vi "TestArrow.vi"() -> ()   [LabVIEW 2018]
uses:
  <vilib>/userdefined/High Color/IMAQdx.ctl
  <vilib>/vision/driver/NI_Vision_Acquisition_Software.lvlib
  <resource>/objmgr/imaqdx.rc
panel:
  in  "Slide":dbl(slide) scale=-1.0..1.0
  out "x-y":u32
  in  "stop":bool
  out "Image":T1(plugin-control)
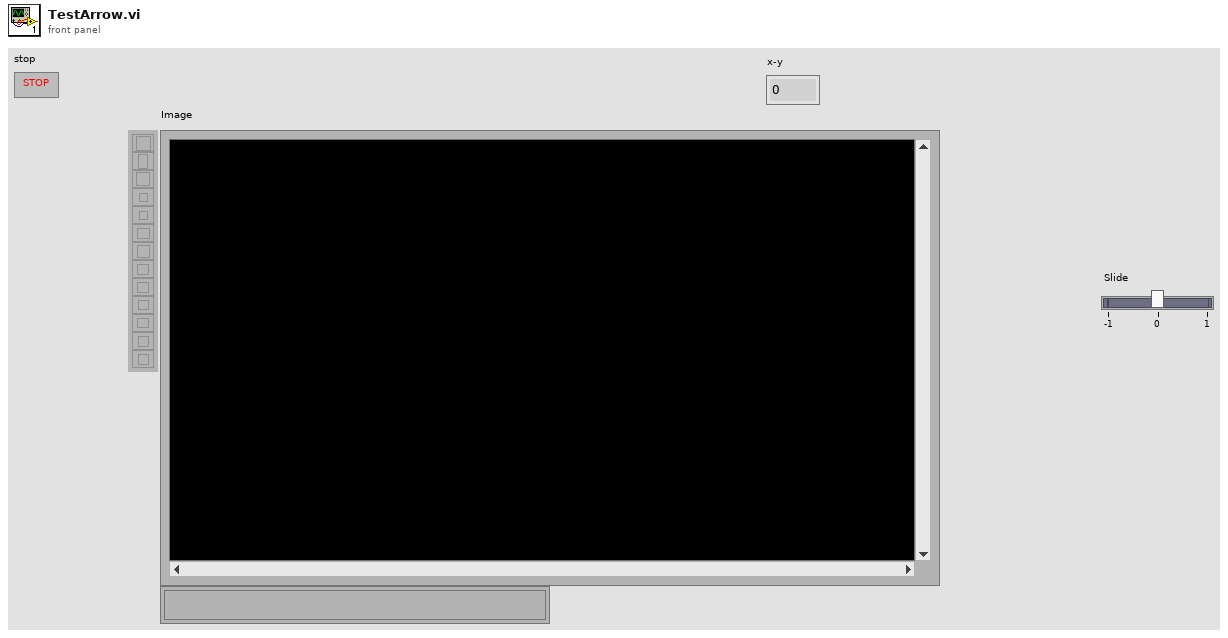
[diagram p1: front panel]
types:
  T1 = typedef "IMAQ Image.ctl" = refnum<image>
  T2 = typedef "IMAQdx.ctl" = refnum<k21>
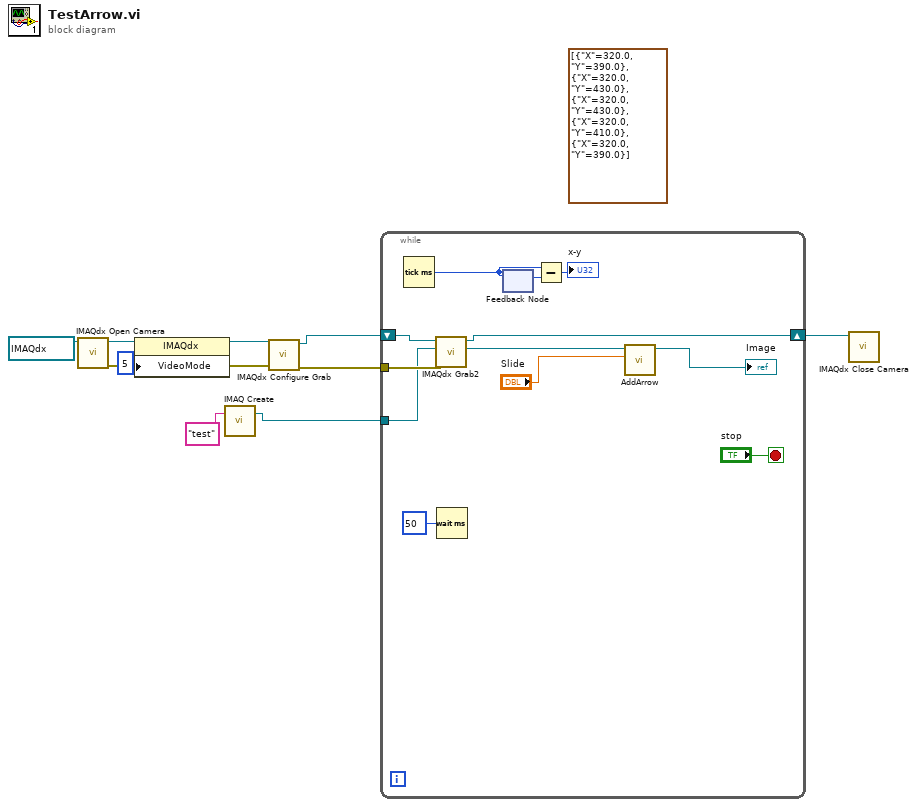
[diagram p0: block diagram]
diagram:
  (unwired) cluster{"X":dbl, "Y":dbl}[] [{"X"=320.0, "Y"=390.0}, {"X"=320.0, "Y"=430.0}, {"X"=320.0, "Y"=430.0}, {"X"=320.0, "Y"=410.0}, {"X"=320.0, "Y"=390.0}] ("Line End Points")
  n1 = call <vilib>:"IMAQdx Open Camera.vi"("Session In"=T2 "cam0") -> ("error out"=w3:errorcluster, "Session Out"=w5:T2)  [unwired: 9 in]
  n2 = property class="IMAQdx"(reference=w5, "VideoMode"=u32 5) -> (reference out=w2:T2)  [unwired: 1 in, 1 out]
  n3 = call "IMAQ Create"("Image Name"="test") -> ("New Image"=w6:T1)  [unwired: 4 in, 1 out]
  n4 = call <vilib>:"IMAQdx Configure Grab.vi"("error in"=w3, "Session In"=w2) -> ("error out"=w8:errorcluster, "Session Out"=w9:T2)  [unwired: 8 in]
  n5 = while {
    tunnel: w8 -> [w21]
    tunnel: w6 -> [w19]
    shift-right: [w14] -> w7
    shift-left: w9 -> [w22]
    stop <- "stop" stop-if-true
    n6 = Tick Count (ms)() -> (millisecond timer value=w17:u32)
    n7 = call <vilib>:"IMAQdx Grab2.vi"("error in"=w21, "Image In"=w19, "Session In"=w22) -> ("Image Out"=w11:T1, "Session Out"=w14:T2)  [unwired: 5 in, 2 out]
    n8 = Wait (ms)(milliseconds to wait=u32 50) -> ()  [unwired: 1 out]
    n9 = feedback-in #1(w17) -> ()
    n10 = feedback #1() -> (w16:u32)  [unwired: 1 in]
    n11 = Subtract(x=w17, y=w16) -> (x-y=→"x-y":u32)
    n12 = call "AddArrow.vi"("Slide"="Slide", "Refnum in"=w11) -> ("Refnum out"=→"Image":T1)  [unwired: 9 in]
  }
  n13 = call <vilib>:"IMAQdx Close Camera.vi"("Session In"=w7) -> ()  [unwired: 10 in, 1 out]
